vi "HAILO_Main.vi"() -> ()   [LabVIEW 2016]
doc: "This example performs writes and reads on a serial port, as directed by the user. You can press the Write and Read buttons, and change the Read Count, while the example is running.\n\nThe parameters set for the serial port must match the parameters of the connected instrument or device. In this example, the Read Count parameter specifies the number of bytes that the serial port reads. If there were more bytes at the port than the specified number, those bytes would not be read. If there were less bytes at the port than the specified number, you would receive a timeout error.\n\nThis example expands upon the flow control options for XON and XOFF, allowing the user to choose those control characters. Also, the user can enable or disable a termination character. Some devices require a termination character in order to identify the end of command strings. Some devices send a termination character to signify the end of data to be read. This example shows how you can end the Read operation once a termination character is detected in the buffer and/or append a termination character at the end of the Write data."
uses:
  <vilib>/ptbypt/NI_PtbyPt.lvlib
panel:
  in  "3D Display":bool
  out "3D Picture":refnum<vi>(3d-picture)
  out "Connection Status":u16(ring) items=["Connecting....", "BT Connected", "Disconnected"]
  in  "Tab Control":T1(tab)=enum."Basic Data"
  out "Channel":u16
  in  "Device Name":string="HAILO"
  in  "F Shear":dbl[](array[numeric])
  in  "dT desired (ms)":u32=20
  in  "3d Display Display every N":i32=4
  in  "Enable  3D":bool
  out "read buffer":string
  out "Sensor Nodes Returned":i32=384
  out "Sensor Readings":i16[][](array[numeric])=[[-533, -111, 239], [-402, 166, 184], [-184, 154, 29], [-106, 74, 11], [-532, -109, 246], [-398, 164, 175], [-205, 152, 32], [-119, 65, 9], [-529, -110, 242], [-408, 166, 184], [-198, 158, 27], [-108, 61, 6], [-539, -106, 240], [-407, 158, 183], [-191, 156, 28], [-113, 73, 15], [816, -260, 842], [539, 512, 512], [156, 425, 83], [13, 142, -72], [816, -262, 840], [528, 520, 512], [162, 425, 83], [13, 137, -84], [809, -260, 840], [538, 520, 504], [162, 432, 72], [13, 136, -84], [809, -260, 846], [538, 508, 512], [158, 435, 72], [19, 136, -79], [346, -168, 14], [287, -68, 19], [161, -34, 4], [70, -44, -7], [345, -191, 19], [279, -40, 8], [167, -16, 12], [72, -23, 2], [341, -190, 17], [285, -46, 9], [149, -15, 6], [54, -40, -2], [375, -201, 19], [282, -51, 10], [135, -37, 6], [81, -57, -12], [-80, -193, -48], [-73, -136, -12], [-5, -122, -31], [-19, -118, -17], [-118, -187, -48], [-73, -115, -22], [1, -113, -27], [-20, -111, -8], [-99, -184, -40], [-62, -145, -17], [0, -113, -37], [-7, -117, -15], [-126, -184, -50], [-72, -115, -14], [-4, -114, -25], [-29, -116, -14]]
  out "Packet OK?":bool=TRUE
  out "Packets Recieved":i32
  out "dT (ms)":dbl
  out "Shear Force":T2(graph)
  out "Normal Force":T3(graph)
  out "Time":u32=427420
  in  "Zero?":bool
  in  "Stop":bool
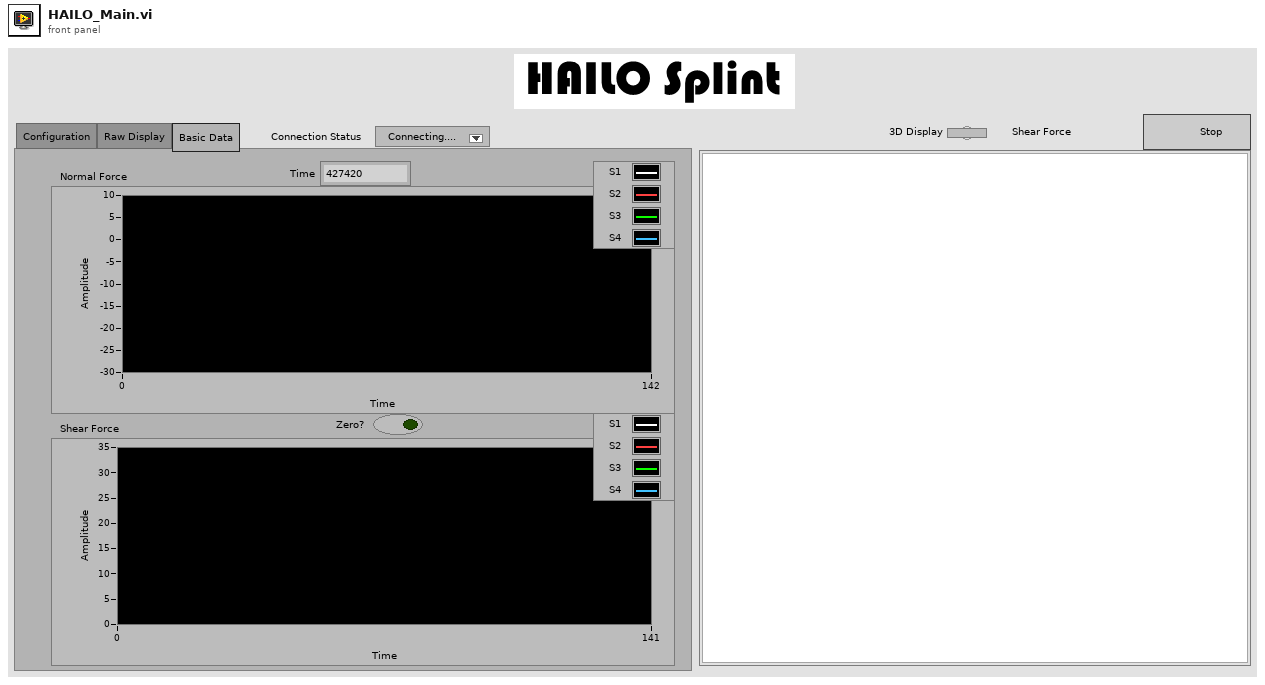
[diagram p1: front panel]
types:
  T1 = enum32{"Configuration", "Raw Display", "Basic Data"}
  T2 = cluster{"F Shear[0]":dbl, "F Shear[1]":dbl, "F Shear[2]":dbl, "F Shear[3]":dbl}
  T3 = cluster{"F Normal[0]":dbl, "F Normal[1]":dbl, "F Normal[2]":dbl, "F Normal[3]":dbl}
  T4 = cluster{"channel":u16, "uuid":string, "service name":string, "service description":string}[]
  T5 = cluster{"channel":u16, "uuid":string, "service name":string, "service description":string}
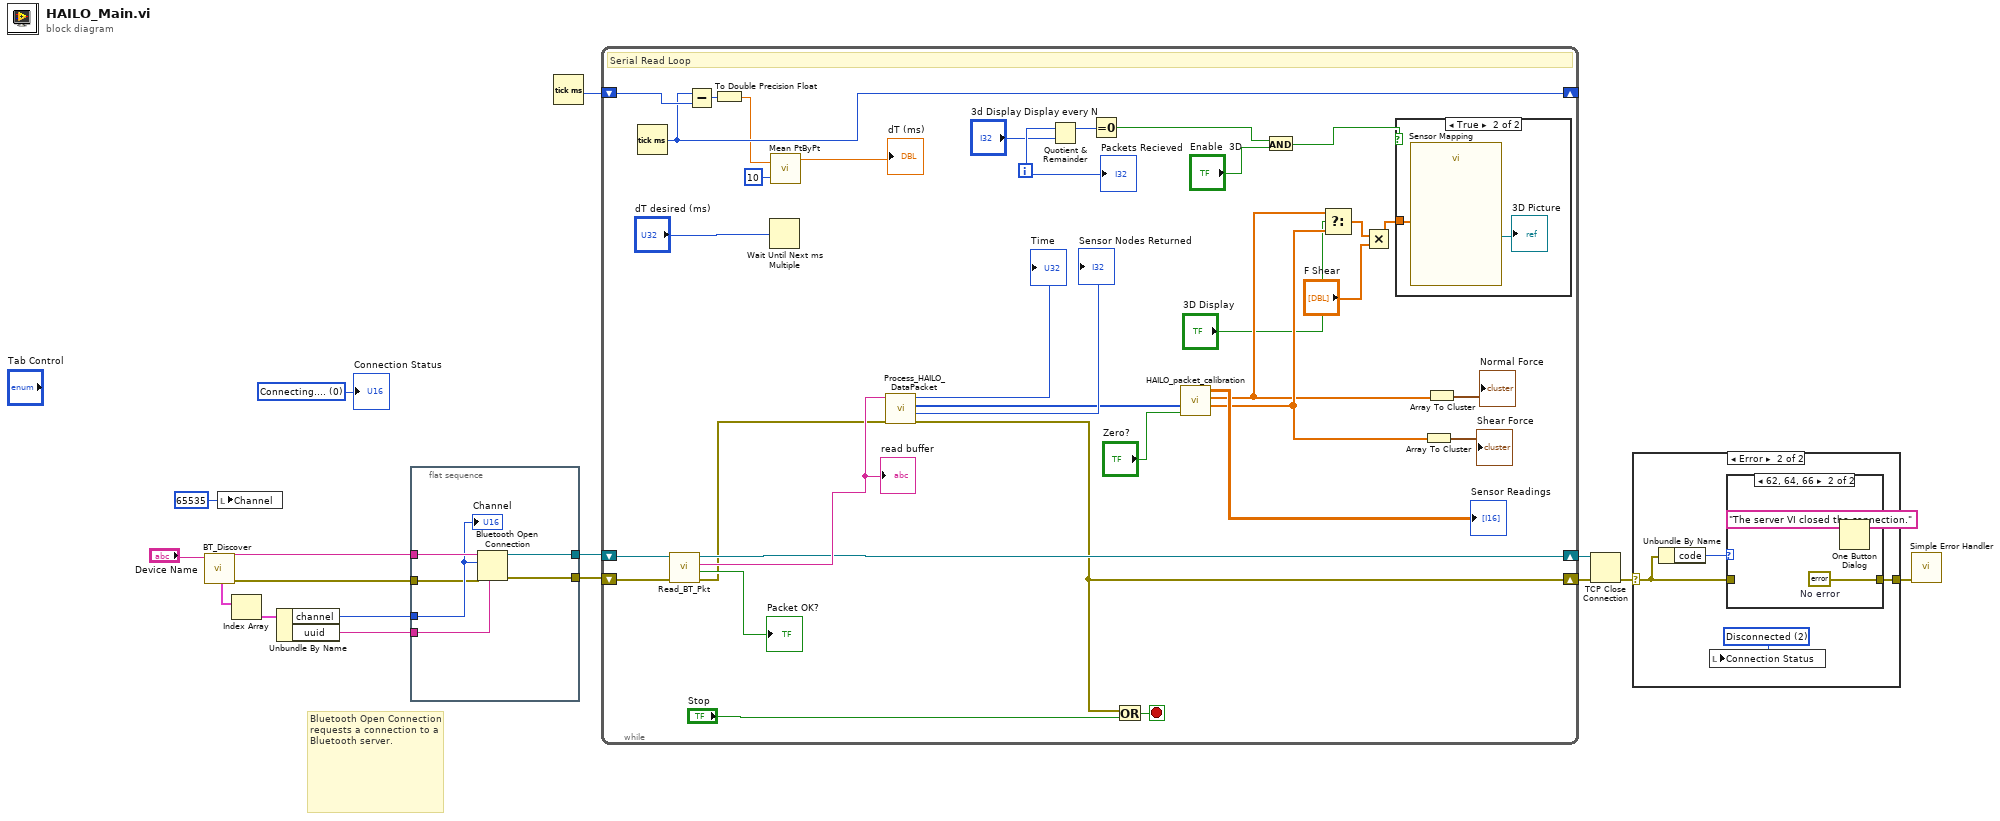
[diagram p0: block diagram]
diagram:
  w2 = u16 0 items=["Connecting....", "BT Connected", "Disconnected"] ("Connection Status")
  # "Bluetooth Open Connection requests a connection to a Bluetooth server."
  n1 = call "BT_Discover.vi"("Device Name"="Device Name") -> ("error out"=w4:errorcluster, "Device Address"=w16:string, "service list"=w15:T4)  [unwired: 6 in, 2 out]
  n2 = local write "Channel"(u16 65535 ("Channel")) -> ()
  n3 = Index Array(array=w15) -> (element=w14:T5)  [unwired: 1 in]
  n4 = Unbundle By Name(w14) -> ("channel"=w11:u16, "uuid"=w13:string)
  n5 = flat-sequence {
    tunnel: w16 -> [w22]
    tunnel: w13 -> [w21]
    tunnel: [w20] -> w12
    tunnel: w11 -> [w19]
    tunnel: [w18] -> w9
    tunnel: w4 -> [w17]
    frame #0 {
      n6 = Bluetooth Open Connection(6:w21, 8:w17, 10:w19, 11:w22) -> (0:w18:errorcluster, 3:w20:refnum<k31>)  [unwired: 1 in]
      "Channel" <- w19
    }
  }
  n7 = Tick Count (ms)() -> (millisecond timer value=w1:u32)
  n8 = while {
    shift-right: [w50] -> w6
    shift-left: w12 -> [w54]
    shift-right: [w47] -> w5
    shift-left: w9 -> [w55]
    shift-right: [w37] -> _
    shift-left: w1 -> [w38]
    i -> [w32]
    stop <- w57 stop-if-true
    # "Serial Read Loop"
    n9 = Tick Count (ms)() -> (millisecond timer value=w37:u32)
    n10 = call "Read_BT_Pkt.vi"("error in"=w55, "connection ID in"=w54) -> ("error out"=w48:errorcluster, "Packet OK?"=→"Packet OK?":bool, "Data"=w53:string, "connection ID out"=w50:refnum<k31>)  [unwired: 6 in]
    "read buffer" <- w53
    n11 = Subtract(x=w37, y=w38) -> (x-y=w34:u32)
    n12 = To Double Precision Float(number=w34) -> (double precision float=w33:dbl)
    n13 = Wait Until Next ms Multiple(millisecond multiple="dT desired (ms)") -> ()  [unwired: 1 out]
    n14 = call <vilib>:"Mean PtByPt.vi"("x"=w33, "sample length"=10) -> ("mean"=→"dT (ms)":dbl)  [unwired: 2 in, 1 out]
    n15 = call "Process_HAILO_DataPacket.vi"("error in (no error)"=w48, "Data Packet"=w53) -> ("error out"=w47:errorcluster, "Sensor Packets Returned"=→"Sensor Nodes Returned":i32, "Sensor Readings (Signed)"=w46:i16[], "Time"=→"Time":u32)  [unwired: 6 in]
    n16 = Quotient & Remainder(x=w32, y="3d Display Display every N") -> (x-y*floor(x/y)=w26:i32)  [unwired: 1 out]
    n17 = Equal To 0?(x=w26) -> (x = 0?=w24:bool)
    n18 = Or(x=w47, y="Stop") -> (x .or. y?=w57:bool)
    n19 = call "HAILO_packet_calibration.vi"("Zero?"="Zero?", "Sensor Readings (Signed)"=w46) -> ("F Shear"=w40:dbl[], "F Normal"=w39:dbl[], "Sensor Readings"=→"Sensor Readings":dbl[][])  [unwired: 7 in]
    n20 = And(x=w24, y="Enable  3D") -> (x .and. y?=w23:bool)
    n21 = Select(t=w39, s="3D Display", f=w40) -> (s? t:f=w29:dbl[])
    n22 = Multiply(x=w29, y="F Shear") -> (x*y=w28:dbl[])
    n23 = case shown="True" w23 {
      tunnel: w28 -> [_ w58]
      frame False {
      }
      frame True {
        n24 = call "Sensor Mapping"("Sensor Values"=w58) -> ("Scene Ref Out"=→"3D Picture":refnum<vi>)  [unwired: 9 in, 1 out]
      }
    }
    n25 = Array To Cluster(array=w40) -> (cluster=→"Shear Force":T2)
    n26 = Array To Cluster(array=w39) -> (cluster=→"Normal Force":T3)
    "Packets Recieved" <- w32
  }
  n27 = TCP Close Connection(connection ID=w6, error in (no error)=w5) -> (error out=w8:errorcluster)  [unwired: 1 in, 1 out]
  n28 = case shown="Error" w8 {
    selector: w8 -> [w60 w63]
    tunnel: [w60 w62] -> w7
    frame No Error {
    }
    frame Error {
      w61 = u16 2 items=["Connecting....", "BT Connected", "Disconnected"] ("Connection Status")
      n29 = Unbundle By Name(w63) -> ("code"=w64:i32)
      n30 = local write "Connection Status"(w61) -> ()
      n31 = case shown="62, 64, 66" w64 {
        tunnel: w63 -> [w65 _]
        tunnel: [w65 w67] -> w62
        frame Default {
        }
        frame 62, 64, 66 {
          w67 = errorcluster {"status"=FALSE, "code"=0, "source"=""}  # No error
          n32 = One Button Dialog(message="The server VI closed the connection." ("Server Closed")) -> ()  [unwired: 1 in, 1 out]
        }
      }
    }
  }
  n33 = call <vilib>:"Simple Error Handler.vi"("error in (no error)"=w7) -> ()  [unwired: 4 in, 5 out]
  "Connection Status" <- w2
